vi "KG get molarity.vi"(7 "Info Cluster":T1, 8 "Fehler (Eingang, kein Fehler)":errorcluster, 10 "pump":u32, 11 "VISA-Ressourcenname":refnum<visa-resource-name>) -> (0 "Fehler (Ausgang)":errorcluster, 1 "Kommando gesendet":string, 2 "molarity":dbl, 3 "VISA-Ressourcenname (Ausgang)":refnum<visa-resource-name>)   [LabVIEW 2020, in "Linearisierung v2.lvlib" / "Gasteiler.lvlib" / "HovaCAL_Interface.lvlib" / "KGN.lvlib" / "get.lvlib"]
uses:
  get.lvlib
  Controls/Info Cluster.ctl
  KGN.lvlib
  Controls/Controls.lvlib
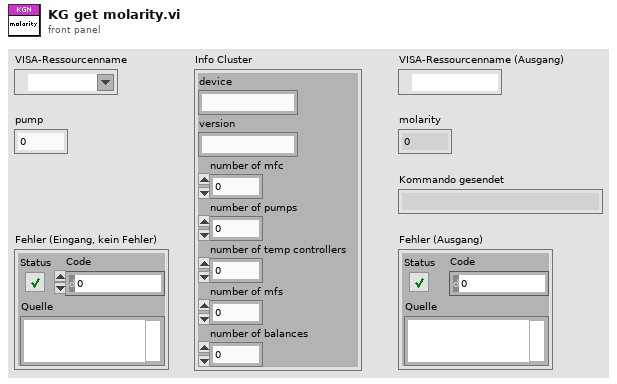
[diagram p1: front panel]
types:
  T1 = typedef "Linearisierung v2.lvlib/Gasteiler.lvlib/HovaCAL_Interface.lvlib/Controls.lvlib/Info Cluster.ctl" = cluster{"device":string, "version":string, "number of mfc":i32, "number of pumps":i32, "number of temp controllers":i32, "number of mfs":i32, "number of balances":i32}
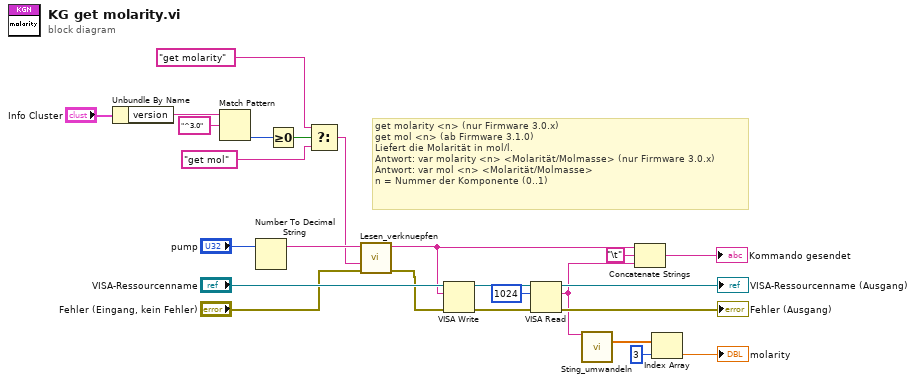
[diagram p0: block diagram]
diagram:
  # "get molarity <n> (nur Firmware 3.0.x)\nget mol <n> (ab Firmware 3.1.0)\nLiefert die Molarität in mol/l.\nAntwort: var molarity <n> <Molarität/Molmasse> (nur Firmware 3.0.x)\nAntwort: var mol <n> <Molarität/Molmasse>\nn = Nummer der Komponente (0..1)"
  n1 = Unbundle By Name("Info Cluster") -> ("version"=w18:string)
  n2 = Match Pattern(string=w18, regular expression="^3.0" ("Regulärer Ausdruck")) -> (offset past match=w16:i32)  [unwired: 1 in, 3 out]
  n3 = Number To Decimal String(number="pump") -> (decimal integer string=w8:string)  [unwired: 1 in]
  n4 = Greater Or Equal To 0?(x=w16) -> (x >= 0?=w15:bool)
  n5 = Select(t="get molarity" ("Schreibpuffer"), s=w15, f="get mol" ("Schreibpuffer")) -> (s? t:f=w7:string)
  n6 = call "Lesen_verknuepfen.vi"("error in (no error)"="Fehler (Eingang, kein Fehler)", "Order"=w7, "param"=w8) -> ("error out"=w10:errorcluster, "Verknüpfter String"=w9:string)  [unwired: 7 in]
  n7 = VISA Write(VISA resource name="VISA-Ressourcenname", write buffer=w9, error in (no error)=w10) -> (VISA resource name out=w25:refnum<visa-resource-name>, error out=w24:errorcluster)  [unwired: 1 out]
  n8 = VISA Read(VISA resource name=w25, byte count=u32 1024 ("Byte-Anzahl"), error in (no error)=w24) -> (VISA resource name out=→"VISA-Ressourcenname (Ausgang)":refnum<visa-resource-name>, read buffer=w2:string, error out=→"Fehler (Ausgang)":errorcluster)  [unwired: 1 out]
  n9 = call "Sting_umwandeln.vi"("Lesepuffer"=w2) -> ("Zahl array"=w6:dbl[])  [unwired: 8 in, 6 out]
  n10 = Concatenate Strings(w9, "\t", w2) -> (→"Kommando gesendet":string)
  n11 = Index Array(array=w6, index=3 ("Index")) -> (element=→"molarity":dbl)
